vi "E364XA Console.vi"() -> ()   [LabVIEW 2010]
uses:
  <vilib>/Instr/_visa.llb/VISA Configure Serial Port (Instr).vi
panel:
  in  "Serial Configuration":T1={"Baud Rate"=9600, "Parity"=0, "Data Bits"=8, "Stop Bits"=20, "Flow Control"=0} {"Flow Control" items=["None", "XON/XOFF", "RTS/CTS", "XON/XOFF & RTS/CTS", "DTR/DSR", "XON/XOFF & DTR/DSR"]; "Stop Bits" items=["1.0"=10, "1.5"=15, "2.0"=20]; "Data Bits" items=["7"=7, "8"=8]; "Parity" items=["None", "Odd", "Even", "Mark", "Space"]; "Baud Rate" items=["300"=300, "600"=600, "1200"=1200, "2400"=2400, "4800"=4800, "9600"=9600, "19200"=19200]}
  out "Current":dbl
  out "Voltage":dbl
  in  "Read":bool
  in  "Stop":bool
  out "Current":string
  out "Voltage":string
  in  "VISA session":refnum<visa-resource-name>="COM9"
  in  "OFF SW":bool
  out "OFF":bool
  in  "ON SW":bool
  out "ON":bool
  out "error out":errorcluster
  in  "error in (no error)":errorcluster
  # "ExTech Console"
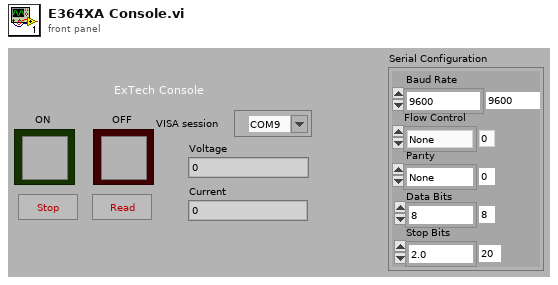
[diagram p1: front panel]
types:
  T1 = cluster{"Baud Rate":u32, "Parity":u16, "Data Bits":u16, "Stop Bits":u16, "Flow Control":u16}
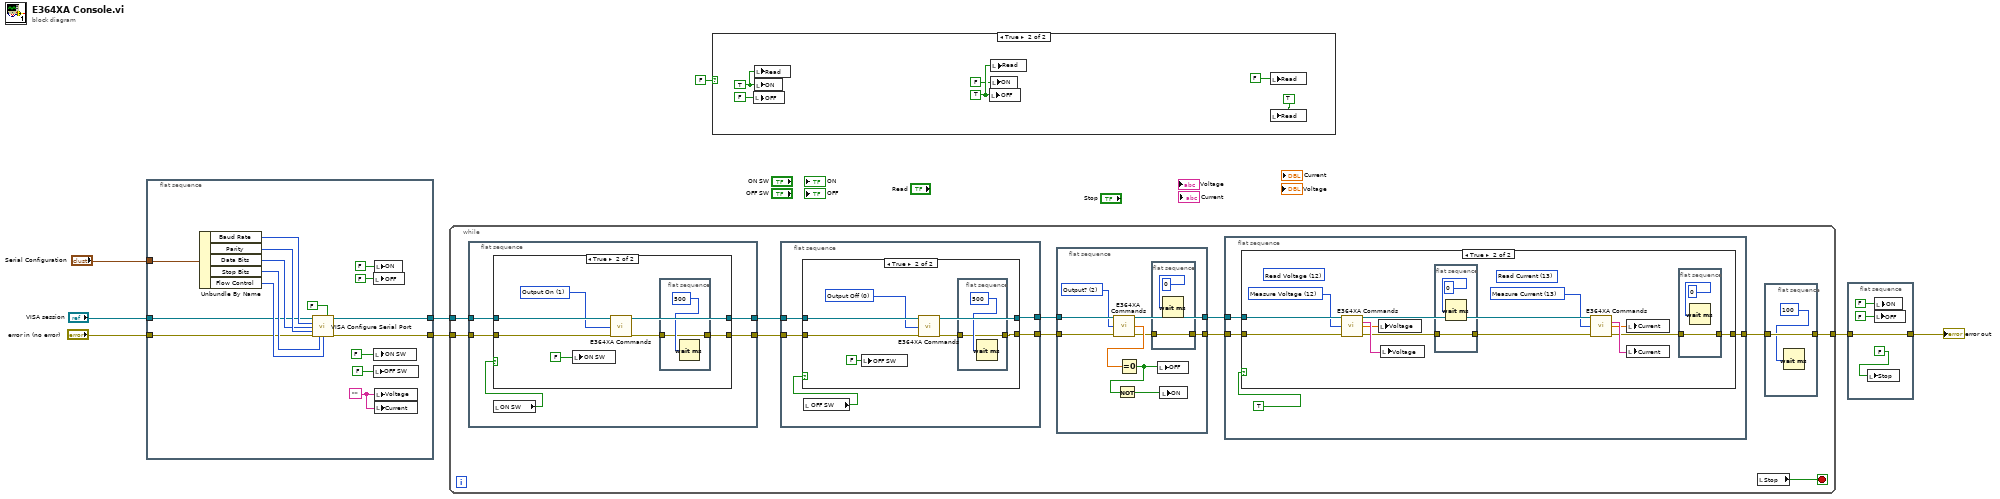
[diagram p0: block diagram]
diagram:
  n1 = flat-sequence {
    tunnel: [w10] -> w5
    tunnel: "error in (no error)" -> [w12]
    tunnel: [w11] -> w3
    tunnel: "VISA session" -> [w13]
    tunnel: "Serial Configuration" -> [w9]
    frame #0 {
      w20 = ""
      n2 = Unbundle By Name(w9) -> ("Baud Rate"=w19:u32, "Parity"=w18:u16, "Data Bits"=w17:u16, "Stop Bits"=w16:u16, "Flow Control"=w15:u16)
      n3 = call-poly "VISA Configure Serial Port"("VISA resource name"=w13, "Enable Termination\nChar (T)"=FALSE, "baud rate (9600)"=w19, "data bits (8)"=w17, "parity (0:none)"=w18, "error in (no error)"=w12, "stop bits (10: 1 bit)"=w16, "flow control (0:none)"=w15) -> ("VISA resource name out"=w11:refnum<visa-resource-name>, "error out"=w10:errorcluster)  [unwired: 6 in]
      n4 = local write "OFF SW"(FALSE) -> ()
      n5 = local write "OFF"(FALSE) -> ()
      n6 = local write "ON SW"(FALSE) -> ()
      n7 = local write "ON"(FALSE) -> ()
      n8 = local write "Voltage"(w20) -> ()
      n9 = local write "Current"(w20) -> ()
    }
  }
  n10 = while {
    tunnel: w3 -> [w30]
    tunnel: w5 -> [w29]
    tunnel: [w31] -> w8
    stop <- w33 stop-if-true
    n11 = flat-sequence {
      tunnel: w30 -> [w91]
      tunnel: w29 -> [w90]
      tunnel: [w89] -> w35
      tunnel: [w88] -> w34
      frame #0 {
        n12 = local read "ON SW"() -> (w87:bool)
        n13 = case shown="True" w87 {
          tunnel: w91 -> [w93 w98]
          tunnel: w90 -> [w92 w99]
          tunnel: [w93 w96] -> w89
          tunnel: [w92 w100] -> w88
          frame False {
          }
          frame True {
            w97 = u16 1 items=["Output Off", "Output On", "Output?", "Voltage Range Low", "Voltage Range High", "Voltage Range?", "Apply 12V, 1.5A", "Apply?", "Voltage 12V", "Voltage?", "Current 1.5A", "Current?", "Measure Voltage", "Measure Current", "Set RS232", "Set Remote Mode", "Set Local Mode", "System Error?", "*IDN?", "*RST", "Instrument Sel?", "Instrument Sel Out 1", "Instrument Sel Out 2", "Display Mode VI", "Display Mode VV", "Display Mode II", "Apply 0V, 0A"] ("Command")
            n14 = local write "ON SW"(FALSE) -> ()
            n15 = call "E364XA Commands.vi"("VISA session"=w98, "Command"=w97, "error in (no error)"=w99) -> ("VISA session out"=w96:refnum<visa-resource-name>, "error out"=w95:errorcluster)  [unwired: 7 in, 4 out]
            n16 = flat-sequence {
              tunnel: [w101] -> w100
              tunnel: w95 -> [w101]
              frame #0 {
                n17 = Wait (ms)(milliseconds to wait=500) -> ()  [unwired: 1 out]
              }
            }
          }
        }
      }
    }
    n18 = flat-sequence {
      tunnel: w35 -> [w75]
      tunnel: w34 -> [w74]
      tunnel: [w73] -> w27
      tunnel: [w72] -> w28
      frame #0 {
        n19 = local read "OFF SW"() -> (w71:bool)
        n20 = case shown="True" w71 {
          tunnel: w75 -> [w77 w84]
          tunnel: w74 -> [w76 w83]
          tunnel: [w77 w82] -> w73
          tunnel: [w76 w80] -> w72
          frame False {
          }
          frame True {
            w79 = u16 0 items=["Output Off", "Output On", "Output?", "Voltage Range Low", "Voltage Range High", "Voltage Range?", "Apply 12V, 1.5A", "Apply?", "Voltage 12V", "Voltage?", "Current 1.5A", "Current?", "Measure Voltage", "Measure Current", "Set RS232", "Set Remote Mode", "Set Local Mode", "System Error?", "*IDN?", "*RST", "Instrument Sel?", "Instrument Sel Out 1", "Instrument Sel Out 2", "Display Mode VI", "Display Mode VV", "Display Mode II", "Apply 0V, 0A"] ("Command")
            n21 = local write "OFF SW"(FALSE) -> ()
            n22 = call "E364XA Commands.vi"("VISA session"=w84, "Command"=w79, "error in (no error)"=w83) -> ("VISA session out"=w82:refnum<visa-resource-name>, "error out"=w81:errorcluster)  [unwired: 7 in, 4 out]
            n23 = flat-sequence {
              tunnel: [w85] -> w80
              tunnel: w81 -> [w85]
              frame #0 {
                n24 = Wait (ms)(milliseconds to wait=500) -> ()  [unwired: 1 out]
              }
            }
          }
        }
      }
    }
    n25 = flat-sequence {
      tunnel: w27 -> [w44]
      tunnel: w28 -> [w43]
      tunnel: [w42] -> w26
      tunnel: [w36] -> w25
      frame #0 {
        w41 = u16 2 items=["Output Off", "Output On", "Output?", "Voltage Range Low", "Voltage Range High", "Voltage Range?", "Apply 12V, 1.5A", "Apply?", "Voltage 12V", "Voltage?", "Current 1.5A", "Current?", "Measure Voltage", "Measure Current", "Set RS232", "Set Remote Mode", "Set Local Mode", "System Error?", "*IDN?", "*RST", "Instrument Sel?", "Instrument Sel Out 1", "Instrument Sel Out 2", "Display Mode VI", "Display Mode VV", "Display Mode II", "Apply 0V, 0A"] ("Command")
        n26 = call "E364XA Commands.vi"("VISA session"=w44, "Command"=w41, "error in (no error)"=w43) -> ("VISA session out"=w42:refnum<visa-resource-name>, "Num Resp"=w40:dbl, "error out"=w37:errorcluster)  [unwired: 7 in, 3 out]
        n27 = Equal To 0?(x=w40) -> (x = 0?=w39:bool)
        n28 = Not(x=w39) -> (.not. x?=w38:bool)
        n29 = flat-sequence {
          tunnel: [w45] -> w36
          tunnel: w37 -> [w45]
          frame #0 {
            n30 = Wait (ms)(milliseconds to wait=0) -> ()  [unwired: 1 out]
          }
        }
        n31 = local write "OFF"(w39) -> ()
        n32 = local write "ON"(w38) -> ()
      }
    }
    n33 = flat-sequence {
      tunnel: [w52] -> w32
      tunnel: w26 -> [w51]
      tunnel: w25 -> [w50]
      frame #0 {
        n34 = case shown="True" TRUE {
          tunnel: [w53 w56] -> w52
          tunnel: w51 -> [_ w66]
          tunnel: w50 -> [w53 w65]
          frame False {
          }
          frame True {
            w60 = u16 13 items=["Output Off", "Output On", "Output?", "Voltage Range Low", "Voltage Range High", "Voltage Range?", "Apply 12V, 1.5A", "Apply?", "Voltage 12V", "Voltage?", "Current 1.5A", "Current?", "Measure Voltage", "Measure Current", "Set RS232", "Set Remote Mode", "Set Local Mode", "System Error?", "*IDN?", "*RST", "Instrument Sel?", "Instrument Sel Out 1", "Instrument Sel Out 2", "Display Mode VI", "Display Mode VV", "Display Mode II", "Apply 0V, 0A"] ("Command")
            w61 = u16 12 items=["Output Off", "Output On", "Output?", "Voltage Range Low", "Voltage Range High", "Voltage Range?", "Apply 12V, 1.5A", "Apply?", "Voltage 12V", "Voltage?", "Current 1.5A", "Current?", "Measure Voltage", "Measure Current", "Set RS232", "Set Remote Mode", "Set Local Mode", "System Error?", "*IDN?", "*RST", "Instrument Sel?", "Instrument Sel Out 1", "Instrument Sel Out 2", "Display Mode VI", "Display Mode VV", "Display Mode II", "Apply 0V, 0A"] ("Command")
            (unwired) u16 13 items=["Standby Mode", "Operating Mode", "Set Voltage", "Set Current", "Set Time", "Set OVP", "Disable OCP", "Enable OCP", "Store", "Recall", "Enable ATS", "Read All Data", "Read Voltage", "Read Current", "Read OCP", "Read OVP", "Read Time", "Read Status"] ("Command")
            (unwired) u16 12 items=["Standby Mode", "Operating Mode", "Set Voltage", "Set Current", "Set Time", "Set OVP", "Disable OCP", "Enable OCP", "Store", "Recall", "Enable ATS", "Read All Data", "Read Voltage", "Read Current", "Read OCP", "Read OVP", "Read Time", "Read Status"] ("Command")
            n35 = call "E364XA Commands.vi"("VISA session"=w66, "Command"=w61, "error in (no error)"=w65) -> ("VISA session out"=w64:refnum<visa-resource-name>, "Response"=w63:string, "Num Resp"=w59:dbl, "error out"=w55:errorcluster)  [unwired: 7 in, 2 out]
            n36 = local write "Voltage"(w59) -> ()
            n37 = local write "Voltage"(w63) -> ()
            n38 = flat-sequence {
              tunnel: [w67] -> w54
              tunnel: w55 -> [w67]
              frame #0 {
                n39 = Wait (ms)(milliseconds to wait=0) -> ()  [unwired: 1 out]
              }
            }
            n40 = call "E364XA Commands.vi"("VISA session"=w64, "Command"=w60, "error in (no error)"=w54) -> ("Response"=w62:string, "Num Resp"=w58:dbl, "error out"=w57:errorcluster)  [unwired: 7 in, 3 out]
            n41 = local write "Current"(w58) -> ()
            n42 = local write "Current"(w62) -> ()
            n43 = flat-sequence {
              tunnel: [w69] -> w56
              tunnel: w57 -> [w69]
              frame #0 {
                n44 = Wait (ms)(milliseconds to wait=0) -> ()  [unwired: 1 out]
              }
            }
          }
        }
      }
    }
    n45 = local read "Stop"() -> (w33:bool)
    n46 = flat-sequence {
      tunnel: w32 -> [w48]
      tunnel: [w48] -> w31
      frame #0 {
        n47 = Wait (ms)(milliseconds to wait=100) -> ()  [unwired: 1 out]
      }
    }
  }
  n48 = case shown="True" FALSE {
    frame False {
    }
    frame True {
      w106 = TRUE
      w108 = TRUE
      n49 = local write "OFF"(FALSE) -> ()
      n50 = local write "Read"(w108) -> ()
      n51 = local write "ON"(w108) -> ()
      n52 = local write "OFF"(w106) -> ()
      n53 = local write "ON"(FALSE) -> ()
      n54 = local write "Read"(w106) -> ()
      n55 = local write "Read"(FALSE) -> ()
      n56 = local write "Read"(TRUE) -> ()
    }
  }
  n57 = flat-sequence {
    tunnel: [w112] -> w7
    tunnel: w8 -> [w112]
    frame #0 {
      n58 = local write "Stop"(FALSE) -> ()
      n59 = local write "OFF"(FALSE) -> ()
      n60 = local write "ON"(FALSE) -> ()
    }
  }
  "error out" <- w7
